vi "Write Name.vi"(8 "error in (no error)":errorcluster, 10 "Name":string="base", 11 "Formatter Config in":refnum<class "Formatter Config.lvclass">) -> (0 "error out":errorcluster, 3 "Formatter Config out":refnum<class "Formatter Config.lvclass">)   [LabVIEW 2015, in "Formatter Config.lvclass"]
uses:
  Formatter Config.lvclass
  Formatter Config.lvclass/Formatter Config.ctl
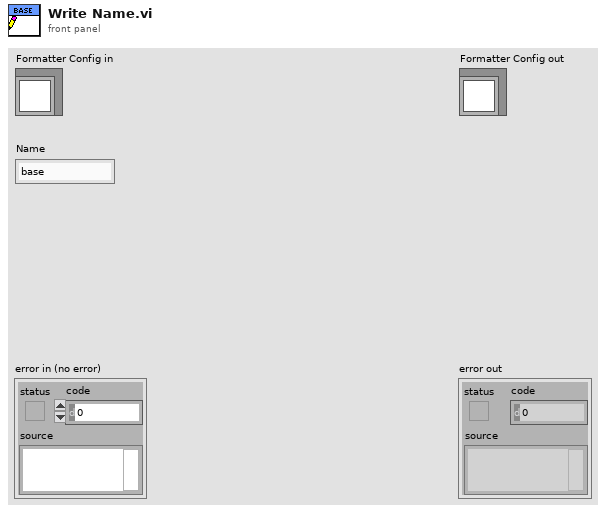
[diagram p1: front panel]
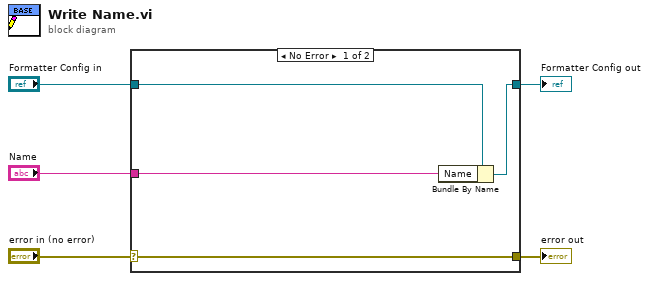
[diagram p0: block diagram]
diagram:
  n1 = case shown="No Error" "error in (no error)" {
    selector: "error in (no error)" -> [w9 w10]
    tunnel: [w9 w10] -> w4
    tunnel: [w7 w11] -> w2
    tunnel: "Formatter Config in" -> [w8 w11]
    tunnel: "Name" -> [w6 _]
    frame No Error {
      n2 = Bundle By Name(cluster=w8, "Name"=w6) -> (w7:refnum<class "Formatter Config.lvclass">)
    }
    frame Error {
    }
  }
  "error out" <- w4
  "Formatter Config out" <- w2
